vi "RunPythonCameraAverage.vi"(10 "filepath":string, 11 "Compiler Settings":T1={"Python Path"=path "", "Main File"="mainscript.py", "Meta File"="metascript.txt", "Aux File"="auxscript.py", "Pre File"="metascript.txt"}) -> (2 "standard error":string, 3 "standard output":string)   [LabVIEW 2019]
uses:
  PulseCompiler/CompilerSettings.ctl
panel:
  in  "error in (no error)":errorcluster
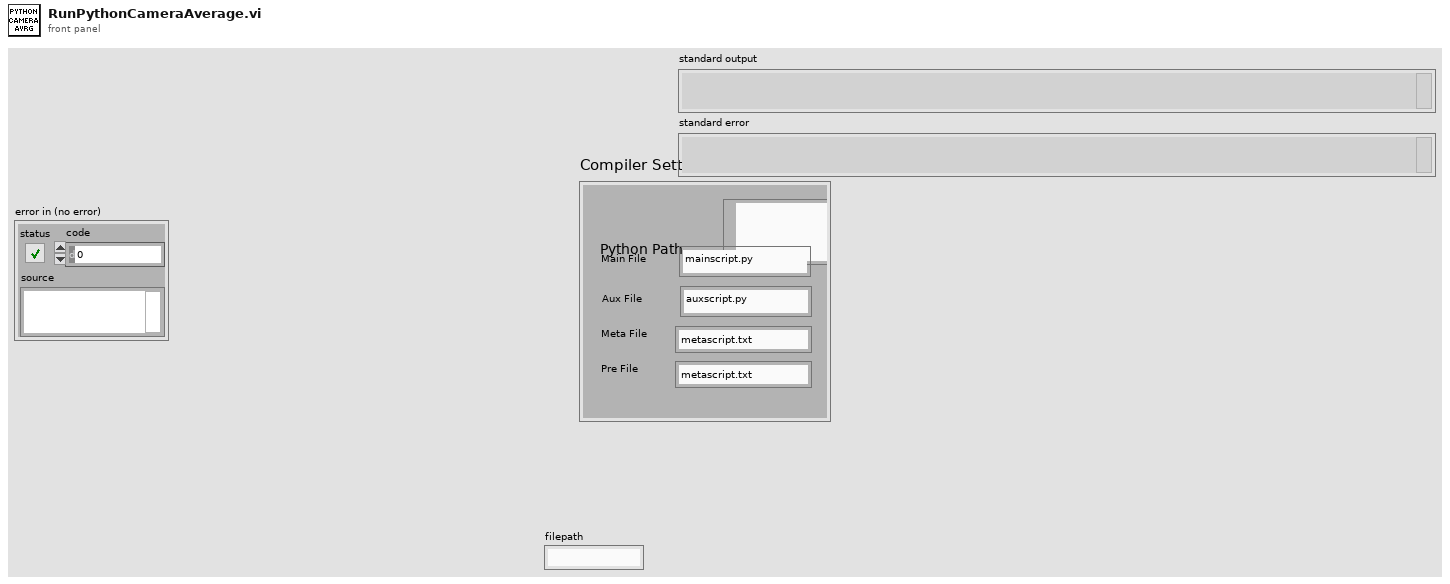
[diagram p1: front panel]
types:
  T1 = typedef "CompilerSettings.ctl" = cluster{"Python Path":path, "Main File":string, "Meta File":string, "Aux File":string, "Pre File":string}
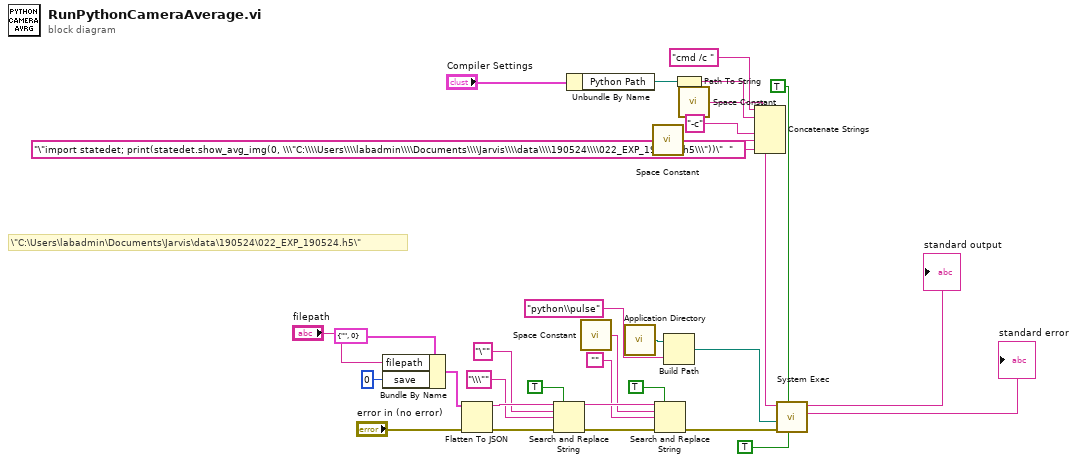
[diagram p0: block diagram]
diagram:
  # "\\\"C:\\Users\\labadmin\\Documents\\Jarvis\\data\\190524\\022_EXP_190524.h5\\\""
  n1 = Bundle By Name(cluster=cluster{"filepath":string, "save":i32} {"filepath"="", "save"=0}, "filepath"="filepath", "save"=0) -> (w11:cluster{"filepath":string, "save":i32})
  n2 = Flatten To JSON(anything=w11, error in (no error)="error in (no error)") -> (JSON string=w23:string, 11:w22:errorcluster)  [unwired: 1 in]
  n3 = Search and Replace String(replace all?=TRUE ("replace all? (F)"), input string=w23, search string="\"", replace string="\\\"" ("replace string (\"\")"), error in=w22) -> (result string=w19:string, error out=w18:errorcluster)  [unwired: 3 in, 2 out]
  n4 = Unbundle By Name("Compiler Settings") -> ("Python Path"=w10:path)
  n5 = call <vilib>:"Space Constant.vi"() -> ("String"=w17:string)
  n6 = call <vilib>:"Application Directory.vi"() -> ("Application Directory"=w25:path)
  n7 = call <vilib>:"Space Constant.vi"() -> ("String"=w5:string)
  n8 = Search and Replace String(replace all?=TRUE ("replace all? (F)"), input string=w19, search string=w17, replace string="", error in=w18) -> (error out=w15:errorcluster)  [unwired: 3 in, 3 out]
  n9 = Build Path(base path=w25, name or relative path="python\\pulse") -> (appended path=w27:path)
  n10 = Path To String(path=w10) -> (string=w9:string)
  n11 = call <vilib>:"Space Constant.vi"() -> ("String"=w6:string)
  n12 = Concatenate Strings("cmd /c " ("string"), w9, w6, "-c" ("string"), w5, "\"import statedet; print(statedet.show_avg_img(0, \\\"C:\\\\Users\\\\labadmin\\\\Documents\\\\Jarvis\\\\data\\\\190524\\\\022_EXP_190524.h5\\\"))\"  " ("string")) -> (w24:string)
  n13 = call <vilib>:"System Exec.vi"("run minimized? (F)"=TRUE, "wait until completion? (T)"=TRUE, "error in (no error)"=w15, "working directory"=w27, "command line"=w24) -> ("standard error"=→"standard error":string, "standard output"=→"standard output":string)  [unwired: 3 in, 2 out]
